vi "ExOptiMosSetupROI.vi"() -> ()   [LabVIEW 2010]
uses:
  Open-Close Hardware/CamHandle.vi
panel:
  out "y dim from camera":u32
  out "x dim from camera":u32
  out "divided by 8":dbl format="%#_16g"
  out "total pixels":u32
  out "y dim":u32
  out "x dim":u32
  out "Exposure Out Mode":u32
  out "Exposure Mode":u32
  in  "Exposure Out":u32(ring)=1 items=["First Row", "All Rows", "Any Row"]
  out "frames":u32=5341
  out "ADC Speed":u32=20000
  out "error out":errorcluster
  in  "error in (no error)":errorcluster
  in  "Timing Mode":u32(ring)=1 items=["N/A"=0, "Timed Mode/Free run"=1, "Internal Trigger"=1792, "Edge Trigger"=2304, "Trigger First"=2048]
  in  "x1":u32=1
  in  "x2":u32=1920
  in  "y1":u32=1
  in  "y2":u32=1080
  in  "x bin":u32=1
  in  "y bin":u32=1
  in  "min block":u32=2
  in  "Num Min Block":u32=5
  # "ExOptiMosSetupROI.vi : This vi setups up 1 ROI (Region Of Interest)."
  # "Note the final ROI must have the pixels \ndivisalbe 8 evenly (whole number, no \nfractional part).\nThis is due to the interfae (not camera)."
  # "Some older versions of the camera firmware didn't support \nBinning. If a labview error occures in error out this migh be \nthe reason"
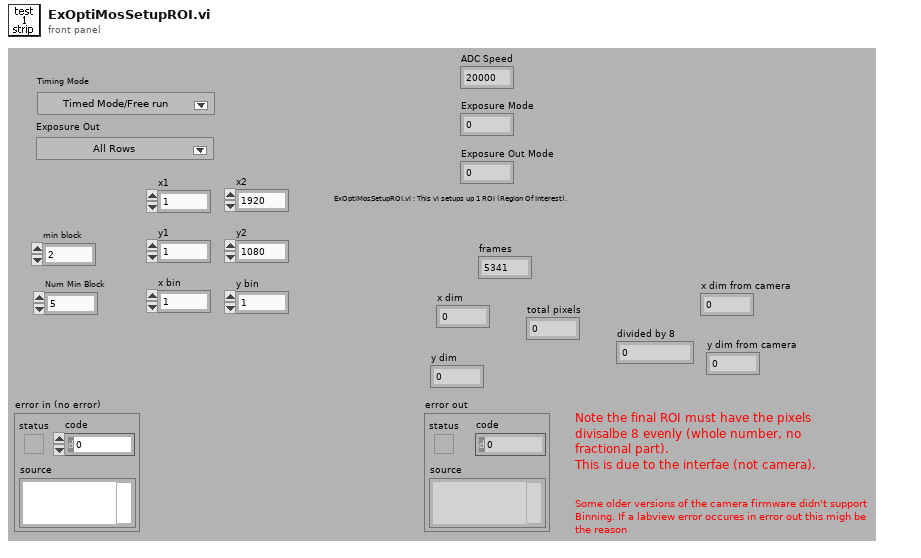
[diagram p1: front panel]
types:
  T1 = cluster{"x1":u32, "x2":u32, "x bin":u32, "y1":u32, "y2":u32, "y bin":u32}
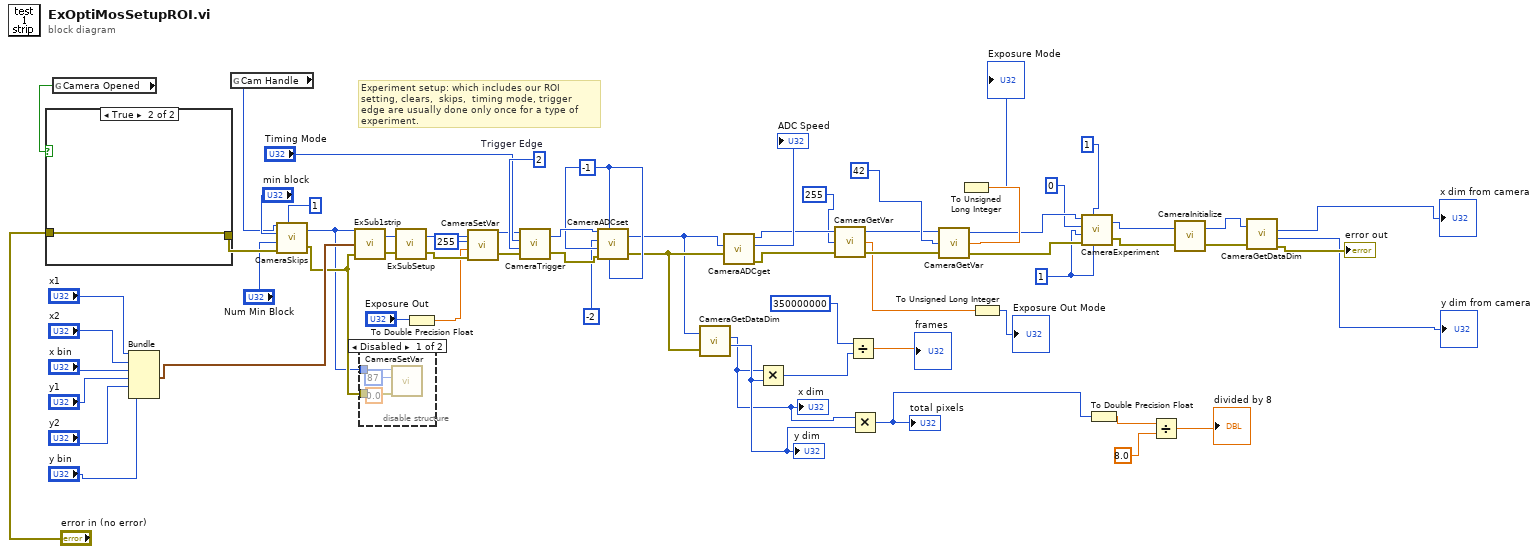
[diagram p0: block diagram]
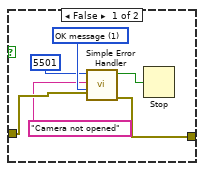
[diagram p3: hidden frame]
diagram:
  w6 = 1
  w61 = -1
  w65 = u32 2  # Trigger Edge
  # "Experiment setup: which includes our ROI setting, clears,  skips,  timing mode, trigger edge are usually done only once for a type of experiment."
  n1 = global read "CamHandle.vi" "Camera Opened"() -> (w64:bool)
  n2 = case shown="True" w64 {
    tunnel: "error in (no error)" -> [w70 w72]
    tunnel: [w69 w72] -> w51
    frame False {
      w71 = u16 1 items=["no dialog", "OK message", "continue or stop message"] ("type of dialog (OK msg:1)")
      n3 = call <vilib>:"Simple Error Handler.vi"("error code (no error:0)"=5501, "error source (\" \")"="Camera not opened", "type of dialog (OK msg:1)"=w71, "error in (no error)"=w70) -> ("error?"=w67:bool, "error out"=w69:errorcluster)  [unwired: 1 in, 3 out]
      n4 = Stop(stop? (T)=w67) -> ()
    }
    frame True {
    }
  }
  n5 = Bundle("x1"="x1", "x2"="x2", "x bin"="x bin", "y1"="y1", "y2"="y2", "y bin"="y bin") -> (w52:T1)  [unwired: 1 in]
  n6 = global read "CamHandle.vi" "Cam Handle"() -> (w46:u32)
  n7 = call <userlib>:"CameraSkips.vi"("Camera Handle"=w46, "Minimum Block Size"="min block", "Number of Minimum blocks"="Num Min Block", "error in"=w51, "Type of Skips"=1) -> ("Camera Handle"=w33:u32, "error out"=w34:errorcluster)
  n8 = call "ExSub1strip.vi"("error in (no error)"=w34, "strip 1"=w52, "Camera Handle"=w33) -> ("error out"=w59:errorcluster, "Camera Handle"=w47:u32)
  n9 = disable-structure shown="Disabled" {
    disable-tunnel: w34 -> [w76 _]
    disable-tunnel: w33 -> [w75 _]
    frame Disabled {
      n10 = call <userlib>:"CameraSetVar.vi"("error in"=w76, "Value"=0.0, "Parameter ID"=u32 87, "Camera Handle"=w75) -> ()  [unwired: 2 out]
    }
    frame Enabled {
    }
  }
  n11 = call "ExSubSetup.vi"("error in (no error)"=w59, "Camera Handle"=w47) -> ("error out"=w32:errorcluster, "Camera Handle"=w30:u32)
  n12 = To Double Precision Float(number="Exposure Out") -> (double precision float=w28:dbl)
  n13 = call <userlib>:"CameraSetVar.vi"("error in"=w32, "Value"=w28, "Parameter ID"=u32 255, "Camera Handle"=w30) -> ("error out"=w31:errorcluster, "CameraHandle"=w29:u32)
  n14 = call <userlib>:"CameraTrigger.vi"("error in"=w31, "Trigger Edge"=w65, "Timing Mode"="Timing Mode", "Camera Handle"=w29) -> ("error out"=w63:errorcluster, "Camera Handle"=w62:u32)
  n15 = call <userlib>:"CameraADCset.vi"("ADC offset"=w61, "Read Out port"=w61, "error in (no error)"=w63, "ADC Gain"=w61, "ADC Speed"=-2, "Camera Handle"=w62) -> ("error out"=w42:errorcluster, "Camera Handle"=w23:u32)
  n16 = call <userlib>:"CameraGetDataDim.vi"("Camera Handle"=w23, "error in"=w42) -> ("Xdim"=w17:u32, "Ydim"=w18:u32)  [unwired: 2 out]
  "x dim" <- w17
  "y dim" <- w18
  n17 = call <userlib>:"CameraADCget.vi"("Camera handle"=w23, "error in (no error)"=w42) -> ("Camera handle"=w24:u32, "ADC Speed"=→"ADC Speed":i32, "error out"=w26:errorcluster)  [unwired: 5 out]
  n18 = Multiply(x=w17, y=w18) -> (x*y=w40:u32)
  n19 = call <userlib>:"CameraGetVar.vi"("error in"=w26, "Parameter ID"=255, "Camera Handle"=w24) -> ("error out"=w25:errorcluster, "Value"=w20:dbl, "Camera Handle"=w22:u32)
  n20 = Divide(x=350000000, y=w40) -> (x/y=→"frames":dbl)
  n21 = Multiply(x=w17, y=w18) -> (x*y=w1:u32)
  "total pixels" <- w1
  n22 = call <userlib>:"CameraGetVar.vi"("error in"=w25, "Parameter ID"=42, "Camera Handle"=w22) -> ("error out"=w14:errorcluster, "Value"=w37:dbl, "Camera Handle"=w10:u32)
  n23 = To Unsigned Long Integer(number=w37) -> (unsigned 32bit integer=→"Exposure Mode":u32)
  n24 = To Unsigned Long Integer(number=w20) -> (unsigned 32bit integer=→"Exposure Out Mode":u32)
  n25 = call <userlib>:"CameraExperiment.vi"("Number of Accumulations"=w6, "Acquire / Focus Flag"=1, "error in"=w14, "Number of Images"=w6, "Exposure (sec)"=0, "Camera Handle"=w10) -> ("error out"=w13:errorcluster, "Camera Handle"=w9:u32)
  n26 = To Double Precision Float(number=w1) -> (double precision float=w2:dbl)
  n27 = Divide(x=w2, y=8.0) -> (x/y=→"divided by 8":dbl)
  n28 = call <userlib>:"CameraInitialize.vi"("error in"=w13, "Camera Handle"=w9) -> ("error out"=w12:errorcluster, "Camera Handle"=w8:u32)
  n29 = call <userlib>:"CameraGetDataDim.vi"("Camera Handle"=w8, "error in"=w12) -> ("Xdim"=→"x dim from camera":u32, "Ydim"=→"y dim from camera":u32, "error out"=→"error out":errorcluster)  [unwired: 1 out]
